vi "addDelayMicroseconds.vi"(8 "error in (no error)":errorcluster, 10 "Microseconds":u16, 11 "Subnet in":refnum<class "Subnet.lvclass">) -> (0 "error out":errorcluster, 3 "Subnet out":refnum<class "Subnet.lvclass">)   [LabVIEW 2016, in "Subnet.lvclass"]
uses:
  Subnet.lvclass
  Subnet.lvclass/Subnet.ctl
  Common_RT_Modbus/IModbus/IModbus.lvclass
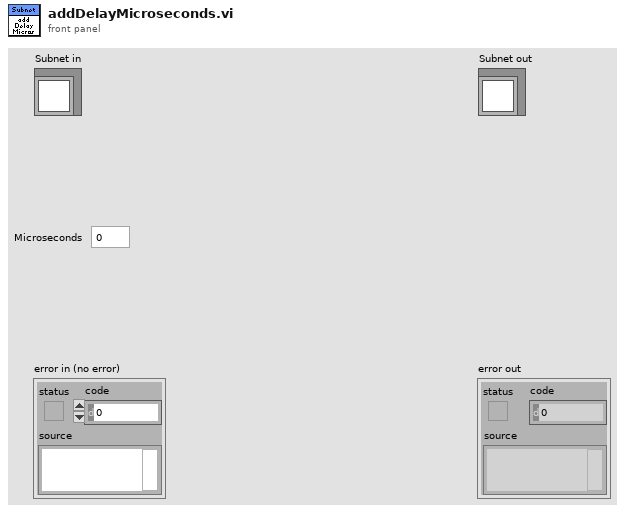
[diagram p1: front panel]
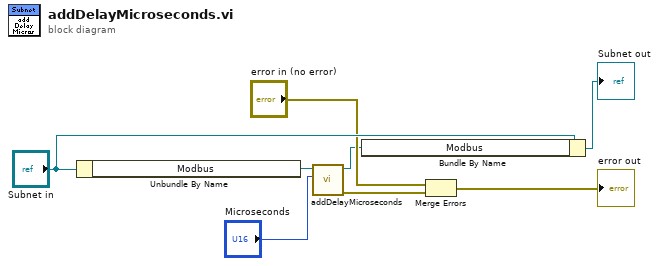
[diagram p0: block diagram]
diagram:
  n1 = Unbundle By Name("Subnet in") -> ("Modbus"=w4:refnum<class "IModbus.lvclass">)
  n2 = call-dynamic "addDelayMicroseconds.vi"("Microseconds"="Microseconds", "IModbus in"=w4) -> ("error out"=w1:errorcluster, "IModbus out"=w3:refnum<class "IModbus.lvclass">)  [unwired: 8 in]
  n3 = Bundle By Name(cluster="Subnet in", "Modbus"=w3) -> (→"Subnet out":refnum<class "Subnet.lvclass">)
  n4 = Merge Errors("error in (no error)", w1) -> (→"error out":errorcluster)
